vi "Progress.vi"() -> ()   [LabVIEW 2018]
panel:
  out "Monitor":T1 {"Elapsed time [s]" format="%#_1g"}
  out "Measure":T2 {"Arduino distance [mm]" format="%#_5g"}
  out "End operation":bool
  out "Measure VS Distance Reference":cluster{dbl[], dbl[]}(graph)
  in  "motor distance":dbl
  out "Progress Output":string
  out "Motor Ready":bool
  out "Communication Acnowledged":bool
  out "error out":errorcluster
  out "Progress":u8(slide) scale=0.0..100.0
  # "Communication\nAcknowledged"
  # "%"
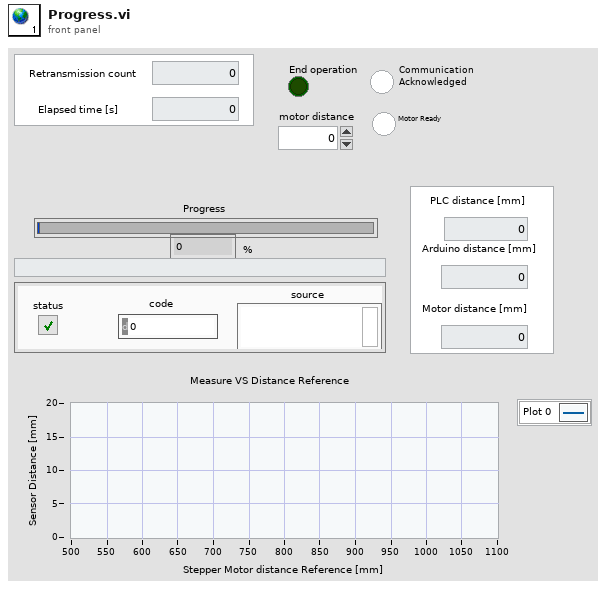
[diagram p1: front panel]
types:
  T1 = cluster{"Elapsed time [s]":dbl, "Retransmission count":dbl}
  T2 = cluster{"PLC distance [mm] ":dbl, "Arduino distance [mm]":dbl, "Motor distance [mm]":dbl}
diagram:
